vi "PID Proportional Control.vi"(0 "Temp":dbl format="%.2f", 7 "Control Parameters":T1={"Setpoint"=50.0, "Control Bandwidth"=4.0, "Integral Time"=30.0, "Int\nON"=TRUE, "Derivative Tme"=0.5, "Der\nON"=TRUE, "Settle Bandwidth"=1.0, "Settle Time"=200.0} {"Settle Time" step=1.0; "Settle Bandwidth" step=0.01; "Derivative Tme" step=0.01; "Integral Time" step=1.0; "Control Bandwidth" step=0.1; "Setpoint" step=0.1}) -> (8 "Proportional Power":dbl format="%.2f")   [LabVIEW 2019]
doc: "This is a Bug C(T) subVI.\n\nThis VI does the PID proportional calculation.\n\nPaul K Dixon\nPhysics 3600\nCSUSB Physics"
uses:
  typedefs/PID control parameters.ctl
panel:
  # "PID\nProportional\nPower\nControl"
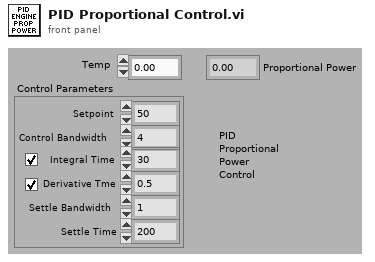
[diagram p1: front panel]
types:
  T1 = typedef "PID control parameters.ctl" = cluster{"Setpoint":dbl, "Control Bandwidth":dbl, "Integral Time":dbl, "Int\nON":bool, "Derivative Tme":dbl, "Der\nON":bool, "Settle Bandwidth":dbl, "Settle Time":dbl}
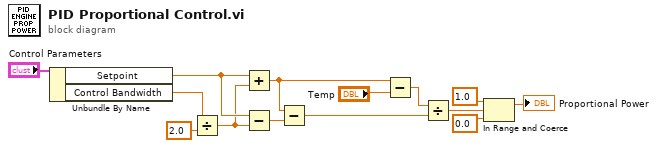
[diagram p0: block diagram]
diagram:
  n1 = Unbundle By Name("Control Parameters") -> ("Setpoint"=w14:dbl, "Control Bandwidth"=w1:dbl)
  n2 = Divide(x=w1, y=2.0) -> (x/y=w13:dbl)
  n3 = Add(x=w14, y=w13) -> (x+y=w10:dbl)
  n4 = Subtract(x=w14, y=w13) -> (x-y=w9:dbl)
  n5 = Subtract(x=w10, y=w9) -> (x-y=w8:dbl)
  n6 = Subtract(x=w10, y="Temp") -> (x-y=w7:dbl)
  n7 = Divide(x=w7, y=w8) -> (x/y=w6:dbl)
  n8 = In Range and Coerce(upper limit=1.0, x=w6, lower limit=0.0) -> (coerced(x)=→"Proportional Power":dbl)  [unwired: 1 out]
